vi "Write Data Start Time.vi"(8 "error in":errorcluster, 10 "Data Start Time":timestamp, 11 "Report Viewer in":refnum<class "Report Viewer.lvclass">) -> (0 "error out":errorcluster, 3 "Report Viewer out":refnum<class "Report Viewer.lvclass">)   [LabVIEW 2019, in "Report Viewer.lvlib" / "Report Viewer.lvclass"]
uses:
  Library/Report Viewer.lvclass
  Custom Controls/Load Method.ctl
  Library/Report Viewer.lvclass/Report Viewer.ctl
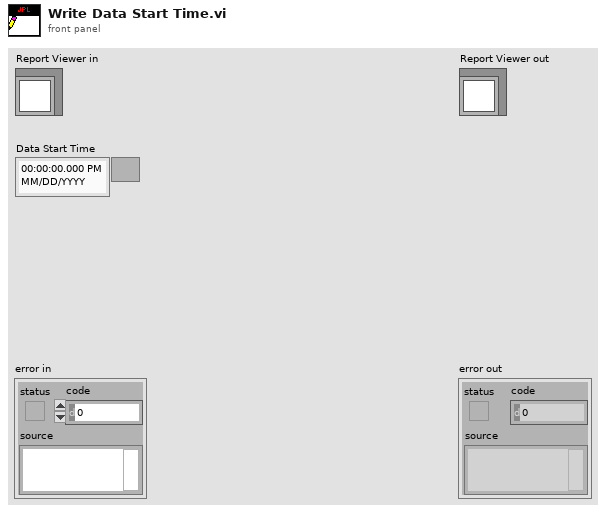
[diagram p1: front panel]
types:
  T1 = typedef "Report Viewer.lvlib/Report Viewer.lvclass/Load Method.ctl" = enum16{"Number of Values", "By Time"}
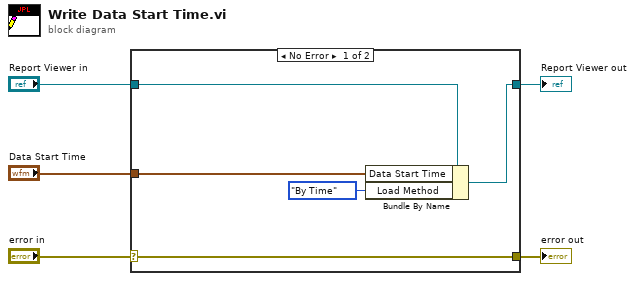
[diagram p0: block diagram]
diagram:
  n1 = case shown="No Error" "error in" {
    selector: "error in" -> [w10 w11]
    tunnel: [w10 w11] -> w4
    tunnel: [w8 w12] -> w2
    tunnel: "Report Viewer in" -> [w9 w12]
    tunnel: "Data Start Time" -> [w7 _]
    frame No Error {
      n2 = Bundle By Name(cluster=w9, "Data Start Time"=w7, "Load Method"=Load_Method."By Time") -> (w8:refnum<class "Report Viewer.lvclass">)
    }
    frame Error {
    }
  }
  "error out" <- w4
  "Report Viewer out" <- w2
